vi "ProcessLidar.vi"(3 "error in":errorcluster, 4 "Direction":dbl[](array[numeric]), 5 "Magnitude":dbl[](array[numeric])) -> (0 "error out":errorcluster, 1 "Lidar Data":cluster{dbl, dbl}[](array[cluster]))   [LabVIEW 2014]
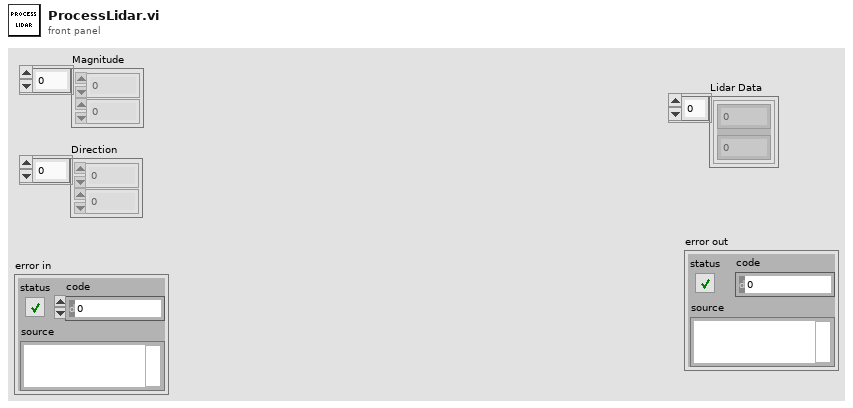
[diagram p1: front panel]
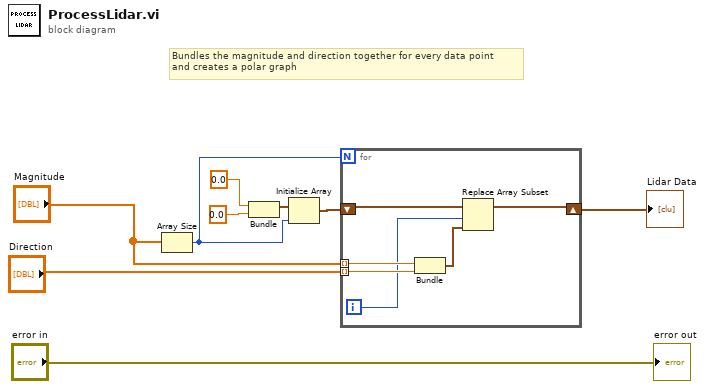
[diagram p0: block diagram]
diagram:
  # "Bundles the magnitude and direction together for every data point\nand creates a polar graph"
  n1 = Array Size(array="Magnitude") -> (size(s)=w5:i32)
  n2 = Bundle(0.0, 0.0) -> (w7:cluster{dbl, dbl})  [unwired: 1 in]
  n3 = Initialize Array(w7, w5) -> (w6:cluster{dbl, dbl}[])
  n4 = for {
    N: w5 -> [_]
    shift-right: [w11] -> w2
    shift-left: w6 -> [w12]
    tunnel: "Magnitude" -> [w15] mode=indexing
    tunnel: "Direction" -> [w14] mode=indexing
    i -> [w13]
    n5 = Bundle(w15, w14) -> (w10:cluster{dbl, dbl})  [unwired: 1 in]
    n6 = Replace Array Subset(array=w12, new element=w10, index=w13) -> (w11:cluster{dbl, dbl}[])
  }
  "Lidar Data" <- w2
  "error out" <- "error in"
